vi "CMD_SUB.vi"(8 "error in (no error)":errorcluster, 10 "Arguments":string[](array[string]), 11 "gScript Interpreter in":refnum<class "gScript Interpreter.lvclass">) -> (0 "error out":errorcluster, 3 "gScript Interpreter out":refnum<class "gScript Interpreter.lvclass">)   [LabVIEW 2017, in "gScript Interpreter.lvclass"]
uses:
  gScript Interpreter.lvclass
  Type Definitions/Memory Cell.ctl
  Type Definitions/Memory Cell Type Enum.ctl
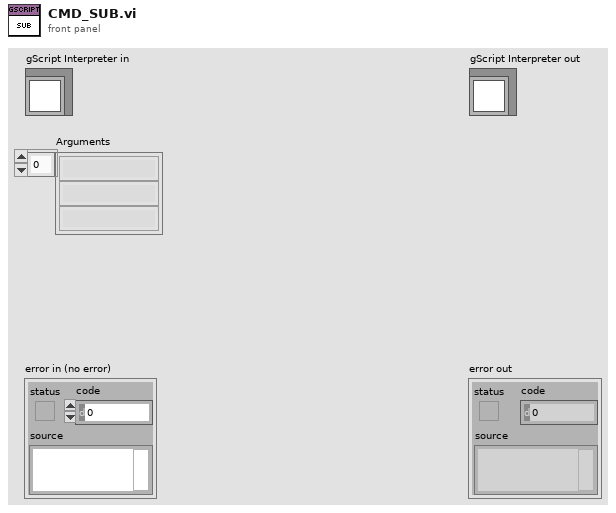
[diagram p1: front panel]
types:
  T1 = typedef "Memory Cell.ctl" = cluster{"type":T2, "x":dbl, "y":dbl, "z":dbl, "w":dbl}
  T2 = typedef "Memory Cell Type Enum.ctl" = enum16{"integer", "float", "vector", "rotation"}
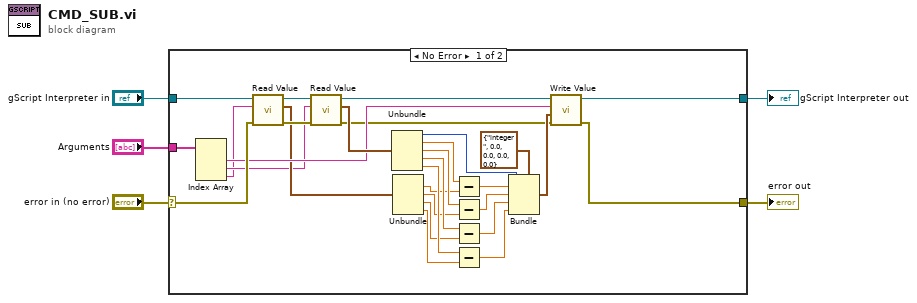
[diagram p0: block diagram]
diagram:
  n1 = case shown="No Error" "error in (no error)" {
    selector: "error in (no error)" -> [w32 w36]
    tunnel: [w9 w36] -> w4
    tunnel: [w10 w35] -> w2
    tunnel: "gScript Interpreter in" -> [w33 w35]
    tunnel: "Arguments" -> [w34 _]
    frame No Error {
      n2 = Index Array(array=w34) -> (element #1=w27:string, element #2=w8:string, element #3=w7:string)  [unwired: 3 in]
      n3 = call-dynamic "Read Value.vi"("error in (no error)"=w32, "String in"=w7, "gScript Interpreter in"=w33) -> ("error out"=w31:errorcluster, "Memory Cell"=w26:T1, "gScript Interpreter out"=w30:refnum<class "gScript Interpreter.lvclass">)  [unwired: 6 in]
      n4 = call-dynamic "Read Value.vi"("error in (no error)"=w31, "String in"=w8, "gScript Interpreter in"=w30) -> ("error out"=w23:errorcluster, "Memory Cell"=w29:T1, "gScript Interpreter out"=w28:refnum<class "gScript Interpreter.lvclass">)  [unwired: 6 in]
      n5 = Unbundle(w29) -> ("type"=w6:T2, "x"=w18:dbl, "y"=w17:dbl, "z"=w16:dbl, "w"=w15:dbl)
      n6 = Unbundle(w26) -> ("x"=w14:dbl, "y"=w13:dbl, "z"=w12:dbl, "w"=w11:dbl)  [unwired: 1 out]
      n7 = Subtract(x=w18, y=w14) -> (x-y=w21:dbl)
      n8 = Subtract(x=w17, y=w13) -> (x-y=w19:dbl)
      n9 = Subtract(x=w16, y=w12) -> (x-y=w20:dbl)
      n10 = Subtract(x=w15, y=w11) -> (x-y=w22:dbl)
      n11 = Bundle(cluster=T1 {"type"=enum."integer", "x"=0.0, "y"=0.0, "z"=0.0, "w"=0.0} ("Memory Cell"), "type"=w6, "x"=w21, "y"=w19, "z"=w20, "w"=w22) -> (w24:T1)
      n12 = call-dynamic "Write Value.vi"("error in (no error)"=w23, "Value"=w24, "Address"=w27, "gScript Interpreter in"=w28) -> ("error out"=w9:errorcluster, "gScript Interpreter out"=w10:refnum<class "gScript Interpreter.lvclass">)  [unwired: 6 in]
    }
    frame Error {
    }
  }
  "error out" <- w4
  "gScript Interpreter out" <- w2
